vi "Lab1 Stopwatch.vi"() -> ()   [LabVIEW 2016]
panel:
  out "Blinker":bool
  in  "Reset Button":bool
  in  "Milliseconds to wait":dbl
  in  "stop":bool
  in  "Pause":bool
  out "Stopwatch":dbl(knob) scale=0.0..10.0
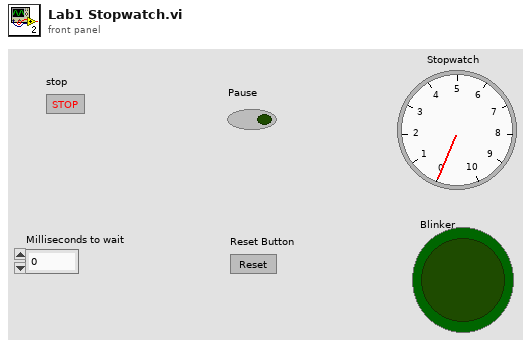
[diagram p1: front panel]
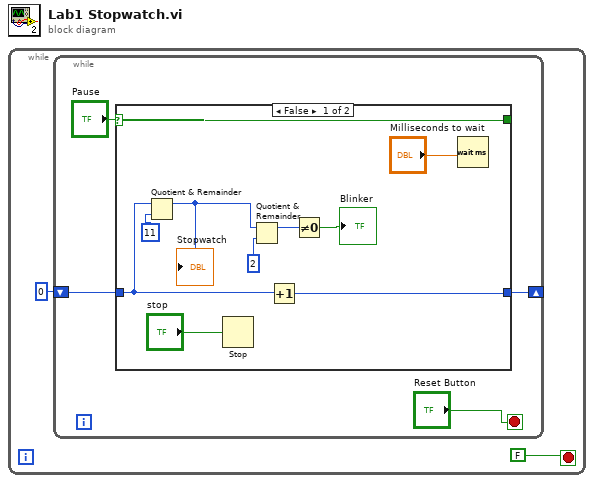
[diagram p0: block diagram]
diagram:
  n1 = while {
    stop <- FALSE stop-if-true
    n2 = while {
      shift-right: [w3] -> _
      shift-left: 0 -> [w4]
      stop <- "Reset Button" stop-if-true
      n3 = case shown="False" "Pause" {
        selector: "Pause" -> [w11 w18]
        tunnel: w4 -> [w8 w17]
        tunnel: [w9 w17] -> w3
        tunnel: [w11 w18] -> _
        frame False {
          n4 = Quotient & Remainder(x=w8, y=11) -> (x-y*floor(x/y)=w7:i32)  [unwired: 1 out]
          "Stopwatch" <- w7
          n5 = Stop(stop? (T)="stop") -> ()
          n6 = Quotient & Remainder(x=w7, y=2) -> (x-y*floor(x/y)=w15:i32)  [unwired: 1 out]
          n7 = Increment(x=w8) -> (x+1=w9:i32)
          n8 = Not Equal To 0?(x=w15) -> (x != 0?=→"Blinker":bool)
          n9 = Wait (ms)(milliseconds to wait="Milliseconds to wait") -> ()  [unwired: 1 out]
        }
        frame True {
        }
      }
    }
  }
